vi "VI Tree - GOLPI.vi"   [LabVIEW 2020, in "GOLPI library.lvlib"]
doc: "Contains all user VI's of the GOLPI library.\n\n---\nGOLPI works only with lv_proc.dll library, which is part of vipm package or should be delivered together with packed library. Placement of this dll is selected in terminal of Start GNU Octave.vi."
uses:
  GOLPI library.lvlib
  Private/Set Variable - polymorph parts/Set String.vi
  Private/Get Variable - polymorph parts/Get String.vi
  LV Process source distribution/Pipe Handle.ctl
  LV Process source distribution/LV Process library.lvlib
  GOLPI reference Type Def.ctl
panel:
  # "SEE DIAGRAM\nFOR VI Tree"
types:
  T1 = typedef "GOLPI library.lvlib/GOLPI reference Type Def.ctl" = cluster{"pipe handle":T2, "fast read timeout [ms]":u32, "fast read settle time [ms]":u32, "fast read to multiple [ms]":u32, "max elements per input line":u32, "slow read timeout [ms]":u32, "stdin double format specifier":string, "max elements per stdout output column":u32, "console mode bitstream":bool, "bitstream first read timeout [ms]":u32, "bitstream read timeout [ms]":u32, "struct transfer possible":bool, "matlab mode":bool}
  T2 = typedef "LV Process library.lvlib/Pipe Handle.ctl" = cluster{"lv_proc.dll file path":path, "process instance handle":u32[], "debug mode":bool, "debug data":cluster{"time":timestamp, "stdin":bool, "data":string}[]}
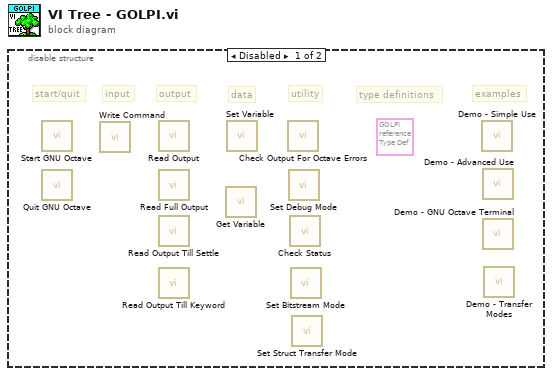
[diagram p0: block diagram]
diagram:
  n1 = disable-structure shown="Disabled" {
    frame Disabled {
      (unwired) T1 {"pipe handle"={"lv_proc.dll file path"=path "", "process instance handle"=[], "debug mode"=FALSE, "debug data"=[]}, "fast read timeout [ms]"=500, "fast read settle time [ms]"=10, "fast read to multiple [ms]"=1, "max elements per input line"=100, "slow read timeout [ms]"=5000, "stdin double format specifier"="%_16e", "max elements per stdout output column"=100, "console mode bitstream"=FALSE, "bitstream first read timeout [ms]"=0, "bitstream read timeout [ms]"=0, "struct transfer possible"=FALSE, "matlab mode"=FALSE} ("GOLPI ref.")
      # "type definitions"
      # "data"
      # "utility"
      # "examples"
      # "output"
      # "input"
      # "start/quit"
      n2 = call "Start GNU Octave.vi"() -> ()  [unwired: 12 in, 4 out]
      n3 = call "Quit GNU Octave.vi"() -> ()  [unwired: 10 in, 2 out]
      n4 = call "Write Command.vi"() -> ()  [unwired: 10 in, 2 out]
      n5 = call "Read Output.vi"() -> ()  [unwired: 8 in, 4 out]
      n6 = call "Read Full Output.vi"() -> ()  [unwired: 8 in, 4 out]
      n7 = call "Read Output Till Settle.vi"() -> ()  [unwired: 8 in, 4 out]
      n8 = call "Read Output Till Keyword.vi"() -> ()  [unwired: 8 in, 4 out]
      n9 = call-poly "Get Variable.vi"() -> ()  [unwired: 9 in, 3 out]
      n10 = call-poly "Set Variable.vi"() -> ()  [unwired: 10 in, 2 out]
      n11 = call "Check Output For Octave Errors.vi"() -> ()  [unwired: 11 in, 1 out]
      n12 = call "Set Debug Mode.vi"() -> ()  [unwired: 8 in, 4 out]
      n13 = call "Check Status.vi"() -> ()  [unwired: 9 in, 3 out]
      n14 = call "Set Bitstream Mode.vi"() -> ()  [unwired: 10 in, 2 out]
      n15 = call "Set Struct Transfer Mode.vi"() -> ()  [unwired: 9 in, 3 out]
      n16 = call "Demo - Simple Use.vi"() -> ()  [unwired: 12 in]
      n17 = call "Demo - Advanced Use.vi"() -> ()  [unwired: 12 in]
      n18 = call "Demo - GNU Octave Terminal.vi"() -> ()  [unwired: 12 in]
      n19 = call "Demo - Transfer Modes.vi"() -> ()  [unwired: 12 in]
    }
    frame Enabled {
    }
  }
